vi "AgNA_Channels Add.vi"(7 "ChannelNumber":i32=1 format="%.0g", 8 "error in (no error)":errorcluster {"code" format="%.0x"}, 9 "ChannelParameter":string, 10 "ChannelType":string, 11 "instrument handle":refnum<k15>) -> (0 "error out":errorcluster {"code" format="%.0x"}, 2 "Val":i32, 3 "instrument handle out":refnum<k15>)   [LabVIEW 2015]
uses:
  <instrlib>/Agilent NA/Agilent NA.lvlib
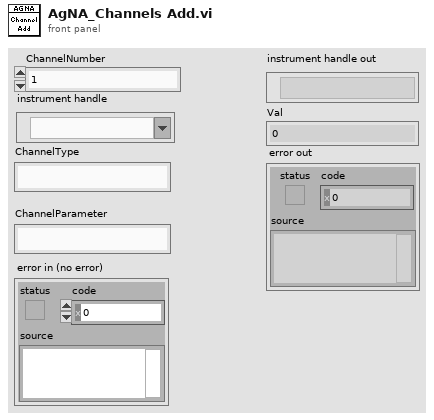
[diagram p1: front panel]
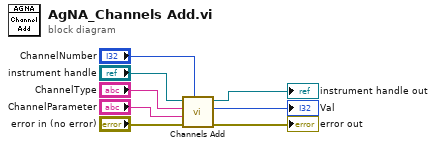
[diagram p0: block diagram]
diagram:
  n1 = call <instrlib>:"Channels Add.vi"("ChannelNumber"="ChannelNumber", "error in (no error)"="error in (no error)", "ChannelParameter"="ChannelParameter", "ChannelType"="ChannelType", "instrument handle"="instrument handle") -> ("error out"=→"error out":errorcluster, "Val"=→"Val":i32, "instrument handle out"=→"instrument handle out":refnum<k15>)  [unwired: 4 in]
